vi "Set Trigger Pulse Width Ns.vi"(8 "error in (no error)":errorcluster, 10 "up_ns":i32, 11 "down_ns":i32) -> (0 "error out":errorcluster)   [LabVIEW 2021, in "vmmso.lvlib"]
doc: "DLL_API void WINAPI SetTriggerPulseWidthNs(int down_ns, int up_ns);"
uses:
  vmmso.lvlib
  vmmso.dll
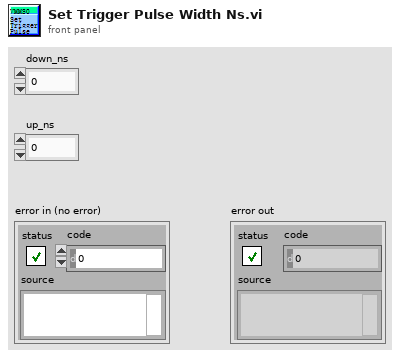
[diagram p1: front panel]
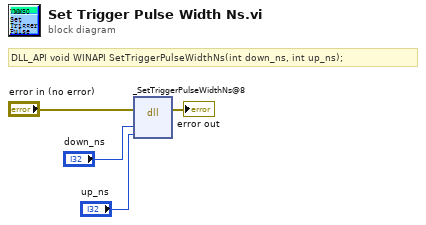
[diagram p0: block diagram]
diagram:
  # "DLL_API void WINAPI SetTriggerPulseWidthNs(int down_ns, int up_ns);"
  n1 = dll-call lib="O:/MSO/library/demo-Labview/vmmso/vmmso.*" fn="_SetTriggerPulseWidthNs@8"(error in="error in (no error)", "down_ns"="down_ns", "up_ns"="up_ns") -> (error out=→"error out":errorcluster)  [unwired: 5 in, 1 out]
